vi "Get Multiple Wheels in Steering Frame.vi"(8 "error in (no error)":errorcluster, 10 "wheel indexes":i32[](array[numeric]), 11 "steering frame in":refnum<class "NI_Robotics_Steering Frame.lvclass">) -> (0 "error out":errorcluster, 1 "found?":bool[](array[boolean]), 2 "wheels":refnum<class "NI_Robotics_Wheel.lvclass">[](array[class]), 3 "steering frame out":refnum<class "NI_Robotics_Steering Frame.lvclass">, 4 "frame angles (rad)":dbl[](array[numeric]), 5 "y positions":dbl[](array[numeric]), 7 "x positions":dbl[](array[numeric]))   [LabVIEW 2017, in "NI_Robotics_Steering Frame.lvclass"]
doc: "Returns the wheels you specify in <B>steering frame in</B> and properties of those wheels. You must manually select the polymorphic instance to use."
uses:
  <vilib>/robotics/Steering/Steering Frame/NI_Robotics_Steering Frame.lvclass
  <vilib>/robotics/Steering/Wheel/NI_Robotics_Wheel.lvclass
  <vilib>/robotics/Steering/Steering Frame/NI_Robotics_Steering Frame.lvclass/NI_Robotics_Steering Frame.ctl
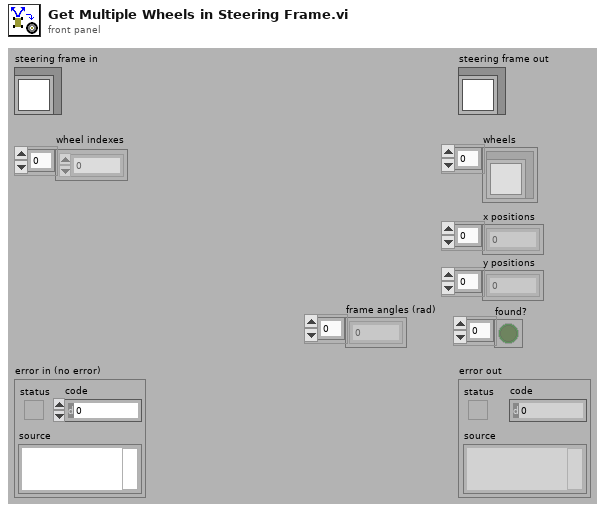
[diagram p1: front panel]
types:
  T1 = typedef "NI_Robotics_Steering Frame.lvclass/Wheel Orientation.ctl" = cluster{"wheel":refnum<class "NI_Robotics_Wheel.lvclass">, "x position":dbl, "y position":dbl, "frame angle (rad)":dbl}
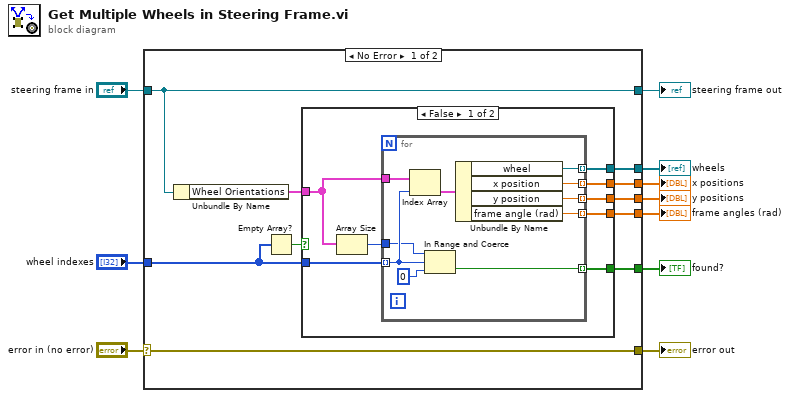
[diagram p0: block diagram]
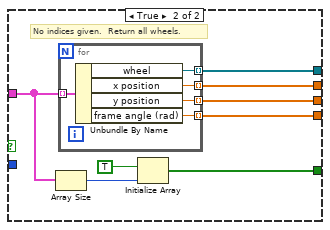
[diagram p2: hidden frame]
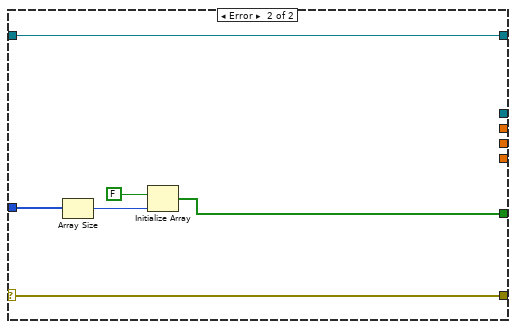
[diagram p3: hidden frame]
diagram:
  n1 = case shown="No Error" "error in (no error)" {
    selector: "error in (no error)" -> [w20 w57]
    tunnel: [w20 w57] -> w9
    tunnel: [w15 w56] -> w7
    tunnel: "steering frame in" -> [w15 w56]
    tunnel: "wheel indexes" -> [w18 w55]
    tunnel: [w19 _] -> w5
    tunnel: [w14 w52] -> w4
    tunnel: [w13 _] -> w3
    tunnel: [w12 _] -> w2
    tunnel: [w11 _] -> w1
    frame No Error {
      n2 = Unbundle By Name(w15) -> ("Wheel Orientations"=w16:T1[])
      n3 = Empty Array?(array=w18) -> (empty?=w17:bool)
      n4 = case shown="False" w17 {
        tunnel: w16 -> [w27 w45]
        tunnel: [w24 w46] -> w19
        tunnel: w18 -> [w28 _]
        tunnel: [w25 w42] -> w14
        tunnel: [w23 w41] -> w13
        tunnel: [w22 w40] -> w12
        tunnel: [w21 w39] -> w11
        frame False {
          n5 = Array Size(array=w27) -> (size(s)=w26:i32)
          n6 = for {
            tunnel: w28 -> [w32] mode=indexing
            tunnel: w27 -> [w38]
            tunnel: w26 -> [w29]
            tunnel: [w30] -> w25 mode=indexing
            tunnel: [w36] -> w24 mode=indexing
            tunnel: [w35] -> w23 mode=indexing
            tunnel: [w34] -> w22 mode=indexing
            tunnel: [w33] -> w21 mode=indexing
            n7 = Index Array(array=w38, index=w32) -> (element=w37:T1)
            n8 = In Range and Coerce(upper limit=w29, x=w32, lower limit=0) -> (In Range?=w30:bool)  [unwired: 1 out]
            n9 = Unbundle By Name(w37) -> ("wheel"=w36:refnum<class "NI_Robotics_Wheel.lvclass">, "x position"=w35:dbl, "y position"=w34:dbl, "frame angle (rad)"=w33:dbl)
          }
        }
        frame True {
          # "No indices given.  Return all wheels."
          n10 = Array Size(array=w45) -> (size(s)=w44:i32)
          n11 = for {
            tunnel: w45 -> [w51] mode=indexing
            tunnel: [w50] -> w46 mode=indexing
            tunnel: [w49] -> w41 mode=indexing
            tunnel: [w48] -> w40 mode=indexing
            tunnel: [w47] -> w39 mode=indexing
            n12 = Unbundle By Name(w51) -> ("wheel"=w50:refnum<class "NI_Robotics_Wheel.lvclass">, "x position"=w49:dbl, "y position"=w48:dbl, "frame angle (rad)"=w47:dbl)
          }
          n13 = Initialize Array(TRUE, w44) -> (w42:bool[])
        }
      }
    }
    frame Error {
      n14 = Array Size(array=w55) -> (size(s)=w54:i32)
      n15 = Initialize Array(FALSE, w54) -> (w52:bool[])
    }
  }
  "error out" <- w9
  "steering frame out" <- w7
  "wheels" <- w5
  "found?" <- w4
  "x positions" <- w3
  "y positions" <- w2
  "frame angles (rad)" <- w1
